vi "提取日志报警参数入列队 (子VI).vi"(10 "索引":i32, 11 "队列输入":refnum<queue>) -> ()   [LabVIEW 2016, in "数据传输系统-05.lvlib"]
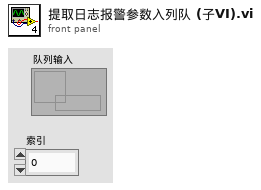
[diagram p1: front panel]
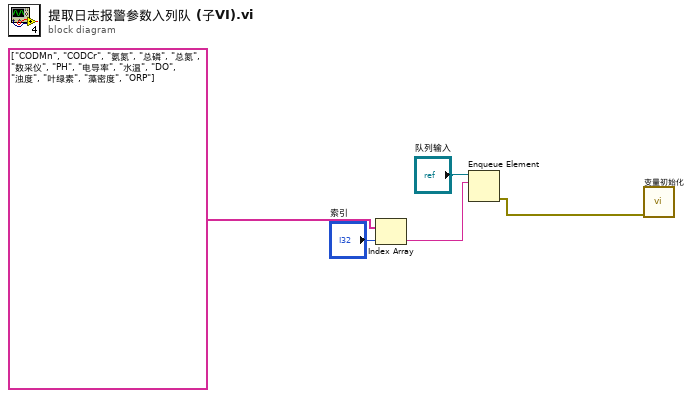
[diagram p0: block diagram]
diagram:
  n1 = Index Array(array=string[] ["CODMn", "CODCr", "氨氮", "总磷", "总氮", "数采仪", "PH", "电导率", "水温", "DO", "浊度", "叶绿素", "藻密度", "ORP"], index="索引") -> (element=w3:string)
  n2 = Enqueue Element(queue="队列输入", element=w3) -> (error out=w1:errorcluster)  [unwired: 2 in, 2 out]
  n3 = call "变量初始化.vi"("错误输入（无错误）"=w1) -> ()  [unwired: 10 in, 1 out]
